vi "Test for reachability.vi"(8 "error in (no error)":errorcluster, 10 "must be directly reachable?":bool, 11 "address":refnum<class "mDNS Hostname Network Address.lvclass">) -> (0 "error out":errorcluster, 2 "found?":bool, 3 "address out":refnum<class "Generic Network Address.lvclass">)   [LabVIEW 2020, in "NI_WFCN.lvlib" / "mDNS Hostname Network Address.lvclass"]
doc: "Determine whether the specified address is reachable."
uses:
  <vilib>/net/WFCN/Addressing/mDNS Hostname Network Address/mDNS Hostname Network Address.lvclass
  e:/builds/penguin/labview/branches/2020/dev/dist/vi.lib/net/WFCN/Addressing/Generic Network Address/Generic Network Address.lvclass
  <vilib>/net/WFCN/Addressing/Generic Network Address/Generic Network Address.lvclass
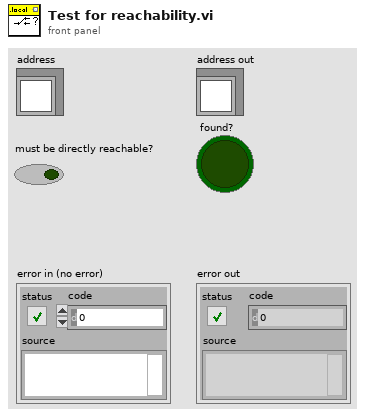
[diagram p1: front panel]
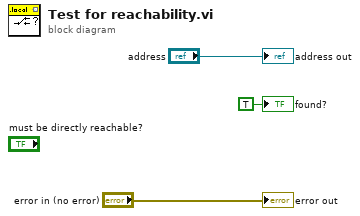
[diagram p0: block diagram]
diagram:
  "error out" <- "error in (no error)"
  "found?" <- TRUE ("found?")
  "address out" <- "address"
